vi "sv_Check for Timeout.vi"(7 "reset":bool, 10 "polling delay [ms]":i32 min=0 max=10000 step=1, 11 "timeout [ms]":i32) -> (2 "elapsed time [ms]":i32, 3 "timeout":bool)   [LabVIEW 2017]
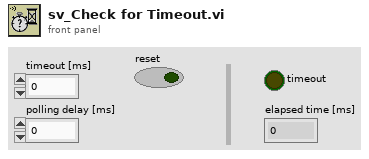
[diagram p1: front panel]
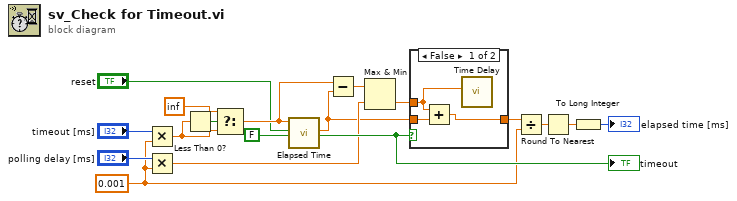
[diagram p0: block diagram]
diagram:
  w6 = 0.001 ("t")
  n1 = Multiply(x="timeout [ms]", y=w6) -> (x*y=w7:dbl)
  n2 = Multiply(x="polling delay [ms]", y=w6) -> (x*y=w9:dbl)
  n3 = Less Than 0?(x=w7) -> (x < 0?=w15:bool)
  n4 = Select(t=inf, s=w15, f=w7) -> (s? t:f=w17:dbl)
  n5 = call "Elapsed Time"("Time Target (s)"=w17, "Reset"="reset", "Auto Reset"=FALSE) -> ("Elapsed Time (s)"=w3:dbl, "Time has Elapsed"=w13:bool)  [unwired: 9 in, 6 out]
  "timeout" <- w13
  n6 = Subtract(x=w17, y=w3) -> (x-y=w18:dbl)
  n7 = Max & Min(x=w18, y=w9) -> (min(x,y)=w14:dbl)  [unwired: 1 out]
  n8 = case shown="False" w13 {
    tunnel: w14 -> [w20 _]
    tunnel: w3 -> [w21 w22]
    tunnel: [w19 w22] -> w2
    frame False {
      n9 = Add(x=w20, y=w21) -> (x+y=w19:dbl)
      n10 = call "Time Delay"("Delay Time (s)"=w20) -> ()  [unwired: 10 in, 1 out]
    }
    frame True {
    }
  }
  n11 = Divide(x=w2, y=w6) -> (x/y=w5:dbl)
  n12 = Round To Nearest(number=w5) -> (nearest integer value=w1:dbl)
  n13 = To Long Integer(number=w1) -> (32bit integer=→"elapsed time [ms]":i32)
